vi "delete_waveform_points.vi"(8 "index":i32, 9 "length":i32=10, 11 "Original Waveform":waveform(dbl)(graph)) -> (0 "New Waveform":waveform(dbl)(graph))   [LabVIEW 2019]
doc: "This VI acquired data is in waveform datatype and can to remove some of the data points."
panel:
  # "Overview:\nThis VI can acquired data is in waveform datatype and also can to remove some of the data \npoints"
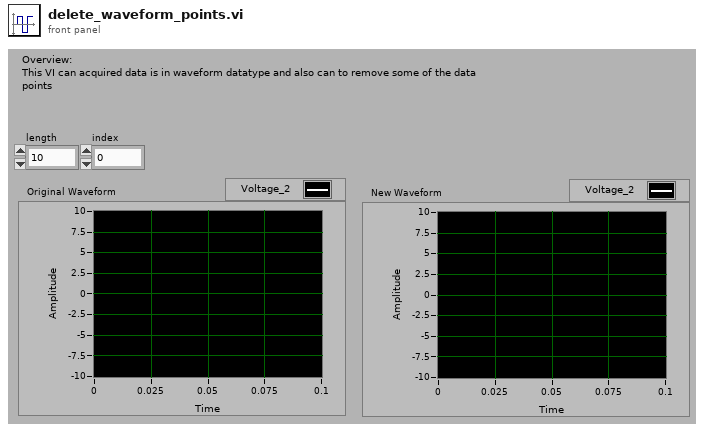
[diagram p1: front panel]
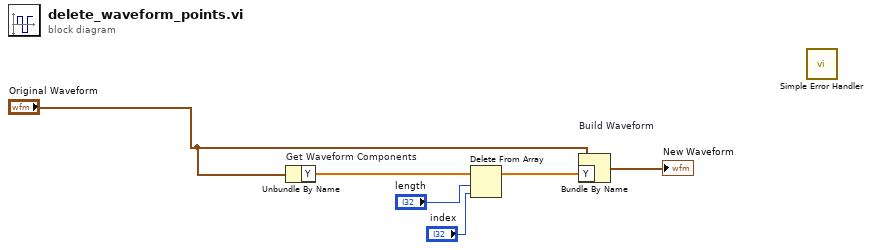
[diagram p0: block diagram]
diagram:
  n1 = Unbundle By Name "Get Waveform Components"("Original Waveform") -> ("Y"=w6:dbl[])
  n2 = Delete From Array "Delete From Array"(array=w6, length="length", index="index") -> (array with subset deleted=w4:dbl[])  [unwired: 1 out]
  n3 = Bundle By Name "Build Waveform"(cluster="Original Waveform", "Y"=w4) -> (→"New Waveform":waveform(dbl))
  n4 = call <vilib>:"Simple Error Handler.vi"() -> ()  [unwired: 5 in, 5 out]
